vi "PointMap_GetAll.vi"(8 "error in (no error)":errorcluster) -> (0 "error out":errorcluster, 1 "All Maps":T1[](array[typedef]), 2 "All Map Names":string[](array[string]))   [LabVIEW 2017, in "PointValueMap.lvlib"]
uses:
  <vilib>/addons/PointValueMap/PointValueMap.lvlib
  <vilib>/addons/PointValueMap/controls/PointMap.ctl
  <vilib>/addons/PointValueMap/controls/PointMapOperations.ctl
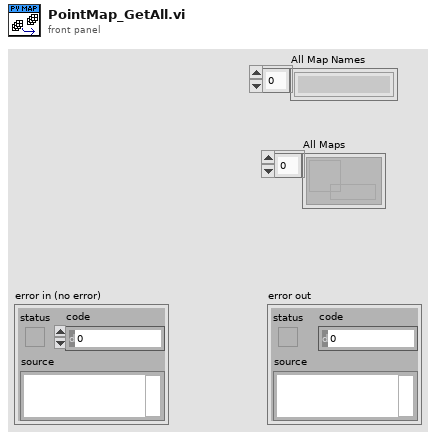
[diagram p1: front panel]
types:
  T1 = typedef "PointValueMap.lvlib/PointMap.ctl" = refnum<data-value>
  T2 = typedef "PointValueMap.lvlib/PointMapOperations.ctl" = enum16{"Initialize", "Create Map", "Update Map", "Get Map", "Get All Maps", "Destroy Map", "Destroy All Maps"}
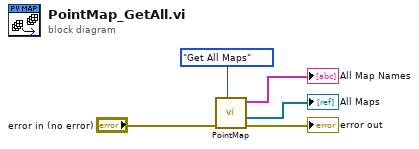
[diagram p0: block diagram]
diagram:
  n1 = call <vilib>:"PointMap.vi"("Operation"=PointMapOperations."Get All Maps", "error in (no error)"="error in (no error)") -> ("error out"=→"error out":errorcluster, "All Maps"=→"All Maps":T1[], "All Map Names"=→"All Map Names":string[])  [unwired: 5 in, 2 out]
